vi "SetInlineActor.vi"(8 "error in (no error)":errorcluster, 10 "Inline (T)":bool=TRUE, 11 "YActor in":refnum<class "YActor.lvclass">) -> (0 "error out":errorcluster, 3 "YActor out":refnum<class "YActor.lvclass">)   [LabVIEW 2021, in "YActor.lvclass"]
doc: "Author: Patriek Bruins\nCompany: Philips\nDepartment: PInS TMA\n\nCopyright © 2017\nAll rights reserved. This VI or any portion thereof may not be used in any application created outside of the Royal Philips company without the express written permission of the author."
uses:
  YActor.lvclass
  YActor.lvclass/YActor.ctl
panel:
  # "Author: Patriek Bruins\nCompany: Philips\nDepartment: PInS TMA\n\nCopyright © 2017\nAll rights reserved. This VI or any portion thereof may not be used in any application created outside of the Royal Philips company without the express written permission of the author."
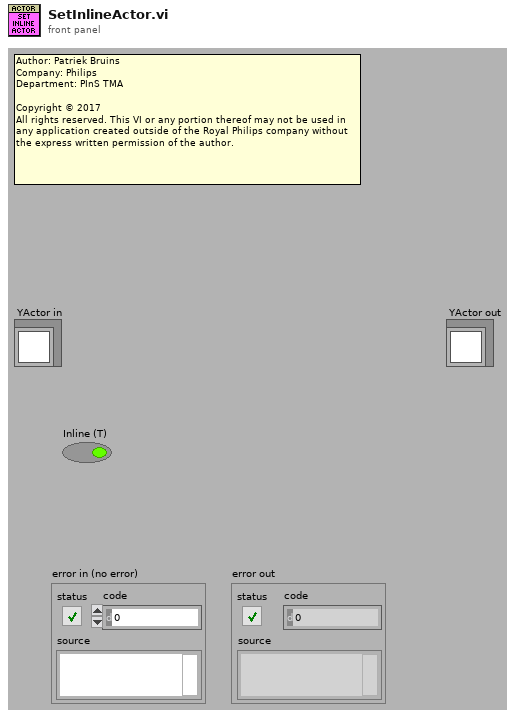
[diagram p1: front panel]
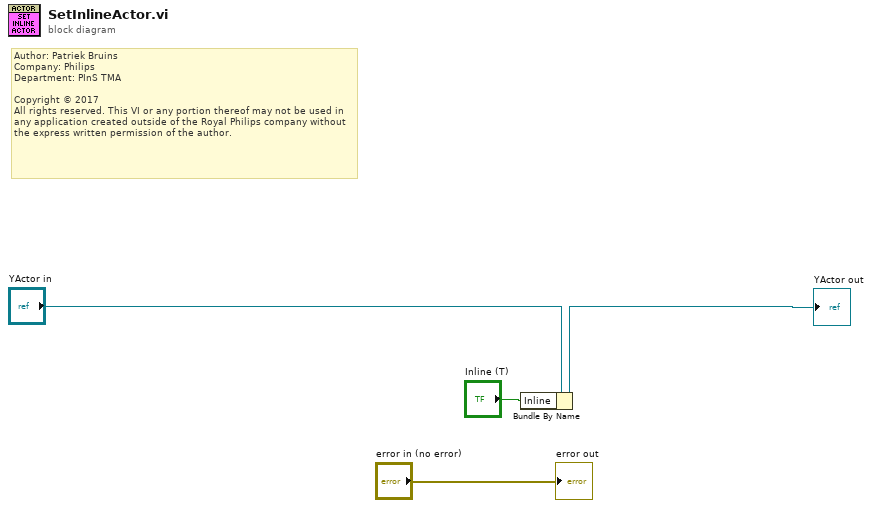
[diagram p0: block diagram]
diagram:
  # "Author: Patriek Bruins\nCompany: Philips\nDepartment: PInS TMA\n\nCopyright © 2017\nAll rights reserved. This VI or any portion thereof may not be used in any application created outside of the Royal Philips company without the express written permission of the author."
  n1 = Bundle By Name(cluster="YActor in", "Inline"="Inline (T)") -> (→"YActor out":refnum<class "YActor.lvclass">)
  "error out" <- "error in (no error)"
